vi "speckle_mask.vi"(6 "SE Size":i32=256, 8 "error in (no error)":errorcluster, 9 "Threshold Multiplier":sgl=2.0, 10 "Image Out":T1, 11 "Image In":T1) -> (0 "error out":errorcluster, 2 "Mask Out":bool[][](array[boolean]), 3 "Image Dst Out":T1)   [LabVIEW 2016]
uses:
  <vilib>/vision/Image Controls.llb/IMAQ Image.ctl
  <vilib>/vision/NI_Vision_Development_Module.lvlib
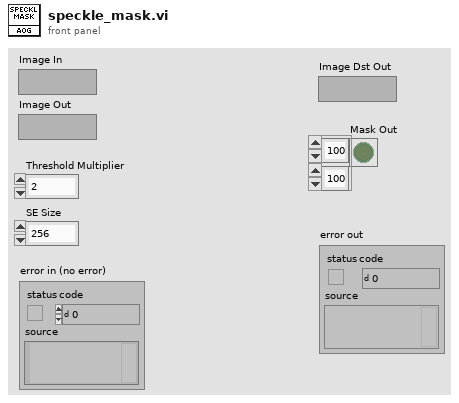
[diagram p1: front panel]
types:
  T1 = typedef "IMAQ Image.ctl" = refnum<image>
  T2 = enum32{"AutoM", "Close", "Dilate", "Erode", "Gradient", "Gradient out", "Gradient in", "Hit miss", "Open", "PClose", "POpen", "Thick", "Thin"}
  T3 = cluster{"histogram":u32[], "Minimal Value":sgl, "Maximal Value":sgl, "Starting Value":sgl, "Interval Width":sgl, "Mean Value":sgl, "Standard  Variation":sgl, "Area (pixels)":i32}
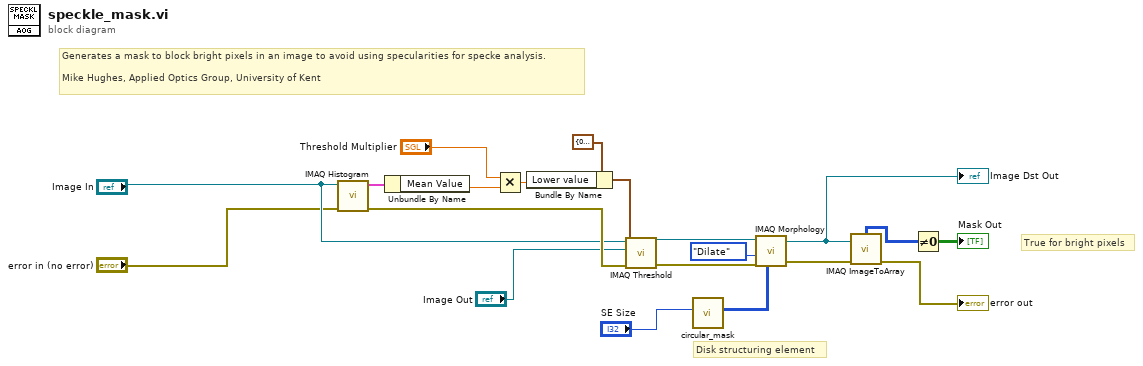
[diagram p0: block diagram]
diagram:
  # "True for bright pixels"
  # "Disk structuring element"
  # "Generates a mask to block bright pixels in an image to avoid using specularities for specke analysis.\n\nMike Hughes, Applied Optics Group, University of Kent"
  n1 = call "IMAQ Histogram"("error in (no error)"="error in (no error)", "Image"="Image In") -> ("error out"=w14:errorcluster, "Histogram Report"=w20:T3)  [unwired: 8 in]
  n2 = Unbundle By Name(w20) -> ("Mean Value"=w19:sgl)
  n3 = Multiply(x="Threshold Multiplier", y=w19) -> (x*y=w16:sgl)
  n4 = Bundle By Name(cluster=cluster{"Lower value":sgl, "Upper value":sgl} {"Lower value"=0.0, "Upper value"=255.0} ("Range"), "Lower value"=w16) -> (w15:cluster{"Lower value":sgl, "Upper value":sgl})
  n5 = call "IMAQ Threshold"("error in (no error)"=w14, "Range"=w15, "Image Dst"="Image Out", "Image Src"="Image In") -> ("error out"=w8:errorcluster, "Image Dst Out"=w12:T1)  [unwired: 6 in]
  n6 = call "circular_mask.vi"("size"="SE Size") -> ("Mask Array"=w11:i16[][])  [unwired: 10 in]
  n7 = call "IMAQ Morphology"("Structuring Element"=w11, "error in (no error)"=w8, "Operation"=T2."Dilate", "Image Src"=w12) -> ("error out"=w6:errorcluster, "Image Dst Out"=w7:T1)  [unwired: 6 in]
  "Image Dst Out" <- w7
  n8 = call "IMAQ ImageToArray"("error in (no error)"=w6, "Image"=w7) -> ("error out"=→"error out":errorcluster, "Image Pixels (U8)"=w2:u8[][])  [unwired: 2 in, 3 out]
  n9 = Not Equal To 0?(x=w2) -> (x != 0?=→"Mask Out":bool[][])
